vi "Global Vars.vi"() -> ()   [LabVIEW 2015]
panel:
  out "Initialising":bool
  out "Aquiring":bool
  out "GPS Lock":bool
  out "GPS Lock Time":dbl
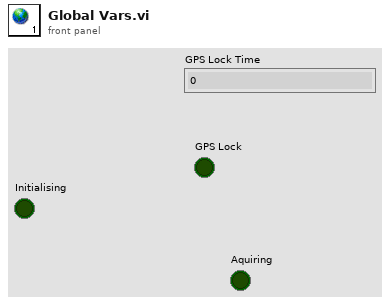
[diagram p1: front panel]
diagram:
